vi "Return Home.vi"(6 "chip select  (1st chip)":enum16{"1st chip", "2nd chip"}(ring), 8 "error in (no error)":errorcluster, 11 "LCD in":refnum<class "Character LCD.lvclass">) -> (0 "error out":errorcluster, 3 "LCD out":refnum<class "Character LCD.lvclass">)   [LabVIEW 2015, in "HD44780 Host.lvlib"]
uses:
  HD44780 Host.lvlib
  Internal/LCD Class/Character LCD.lvclass
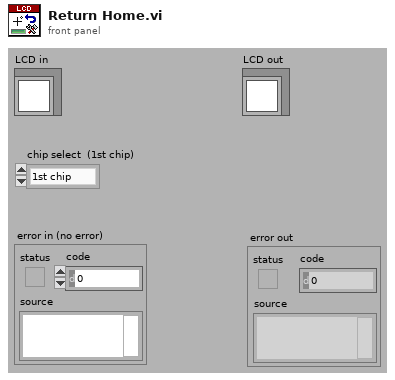
[diagram p1: front panel]
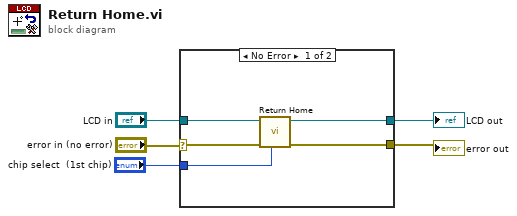
[diagram p0: block diagram]
diagram:
  n1 = case shown="No Error" "error in (no error)" {
    selector: "error in (no error)" -> [w6 w11]
    tunnel: [w7 w11] -> w5
    tunnel: "chip select  (1st chip)" -> [w10 _]
    tunnel: "LCD in" -> [w9 w12]
    tunnel: [w8 w12] -> w1
    frame No Error {
      n2 = call-dynamic "Return Home.vi"("chip select  (1st chip)"=w10, "error in (no error)"=w6, "Character LCD in"=w9) -> ("error out"=w7:errorcluster, "Character LCD out"=w8:refnum<class "Character LCD.lvclass">)  [unwired: 7 in]
    }
    frame Error {
    }
  }
  "error out" <- w5
  "LCD out" <- w1
